vi "Assert Commit 2D Array.vi"() -> ()   [LabVIEW 2015, in "Admin_Actor.lvlib" / "ExcuseNotesHandler.lvclass"]
uses:
  ExcuseNotesHandler.lvclass
  API/_Database/Database.lvclass
  ExcuseNotesHandler.lvclass/ExcuseNotesHandler.ctl
panel:
  out "2D Array":string[][](array[string])
  in  "path":path=path "E:/哈工大竞技机器人队/机器人队管理系统/Database/CRTDatabase.accdb"
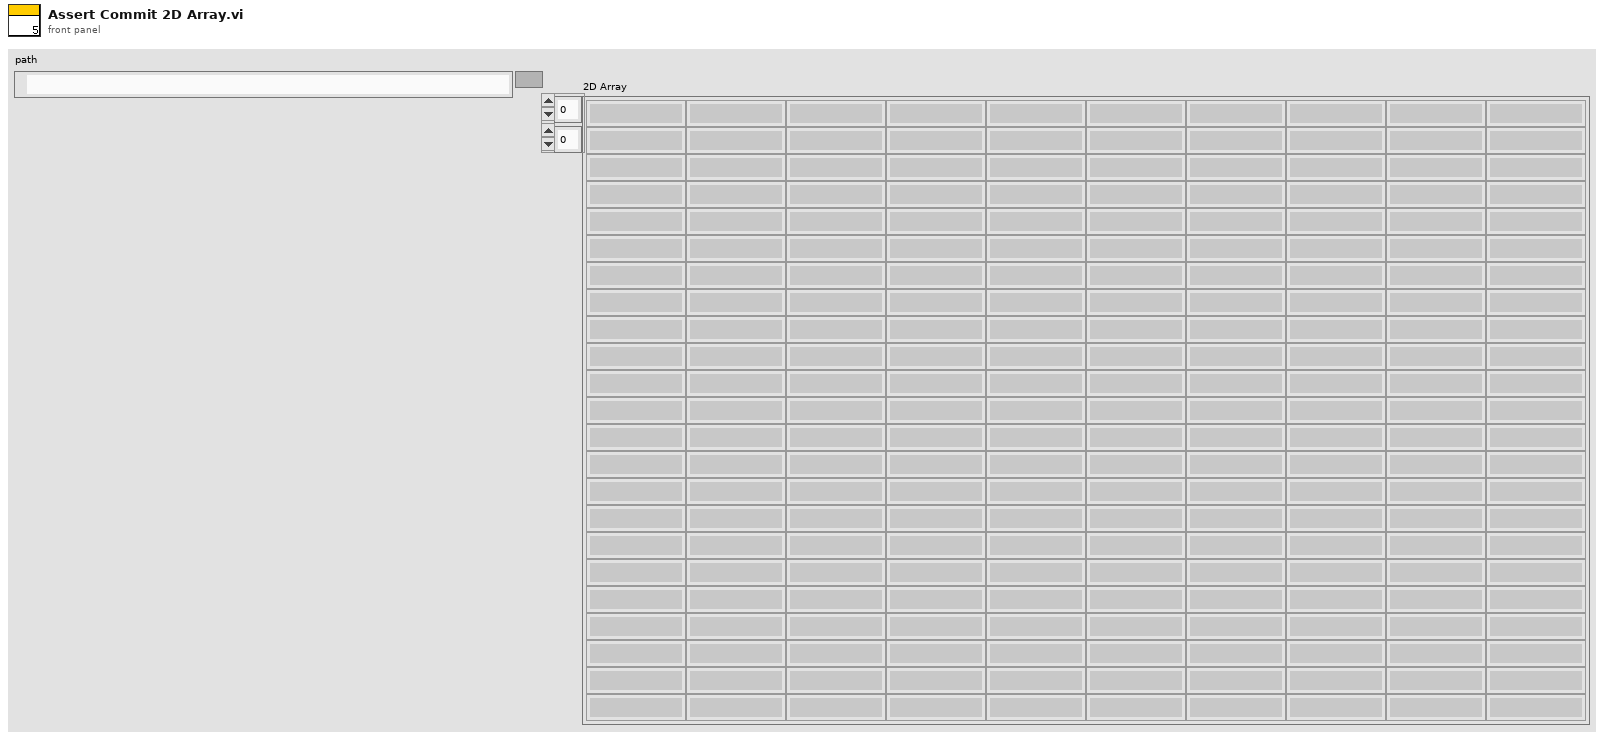
[diagram p1: front panel]
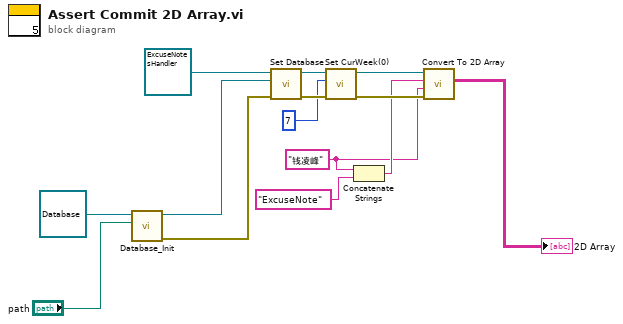
[diagram p0: block diagram]
diagram:
  w2 = "钱凌峰" ("Name")
  n1 = call "Database_Init.vi"("path"="path", "object in"=refnum<class "Database.lvclass"> refnum ("Database")) -> ("error out"=w10:errorcluster, "object out"=w11:refnum<class "Database.lvclass">)  [unwired: 8 in]
  n2 = call "Set Database.vi"("error in (no error)"=w10, "Database"=w11, "ExcuseNotes in"=refnum<class "ExcuseNotesHandler.lvclass"> refnum ("Admin_Actor.lvlib:ExcuseNotes.lvclass")) -> ("error out"=w8:errorcluster, "ExcuseNotes out"=w9:refnum<class "ExcuseNotesHandler.lvclass">)  [unwired: 7 in]
  n3 = call "Set CurWeek(0).vi"("error in (no error)"=w8, "CurWeek(0)"=7, "ExcuseNotesHandler in"=w9) -> ("error out"=w5:errorcluster, "ExcuseNotesHandler out"=w6:refnum<class "ExcuseNotesHandler.lvclass">)  [unwired: 7 in]
  n4 = Concatenate Strings(w2, "ExcuseNote" ("string")) -> (w3:string)
  n5 = call "Convert To 2D Array.vi"("error in (no error)"=w5, "Name"=w2, "TableName"=w3, "ExcuseNotesHandler"=w6) -> ("2D Array"=→"2D Array":string[][])  [unwired: 5 in, 2 out]
